vi "Measurement-IN.vi"(1 "Ctl Refnum 2":refnum<vi>, 2 "Ctl Refnum":refnum<vi>, 8 "error in (no error)":errorcluster, 9 "BSFR":refnum<file>, 10 "Cluster 2":T3, 11 "测试时间":dbl) -> (7 "Cluster":T1)   [LabVIEW 2017]
uses:
  <vilib>/Instr/_visa.llb/VISA Configure Serial Port (Instr).vi
panel:
  out "电抗":dbl
  out "电阻":dbl
  in  "Cluster 3":T2
  in  "高温&低温":u16(ring) items=["低温", "高温"]
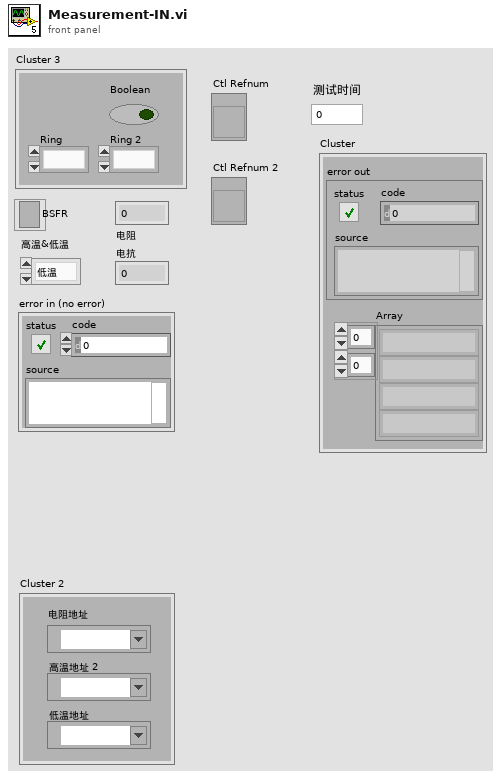
[diagram p1: front panel]
types:
  T1 = cluster{"Array":string[][], "error out":errorcluster}
  T2 = cluster{"Boolean":bool, "Ring":u16, "Ring 2":u16}
  T3 = cluster{"电阻地址":refnum<visa-resource-name>, "低温地址":refnum<visa-resource-name>, "高温地址 2":refnum<visa-resource-name>}
  T4 = cluster{"Array 2":string[][], "error out":errorcluster}
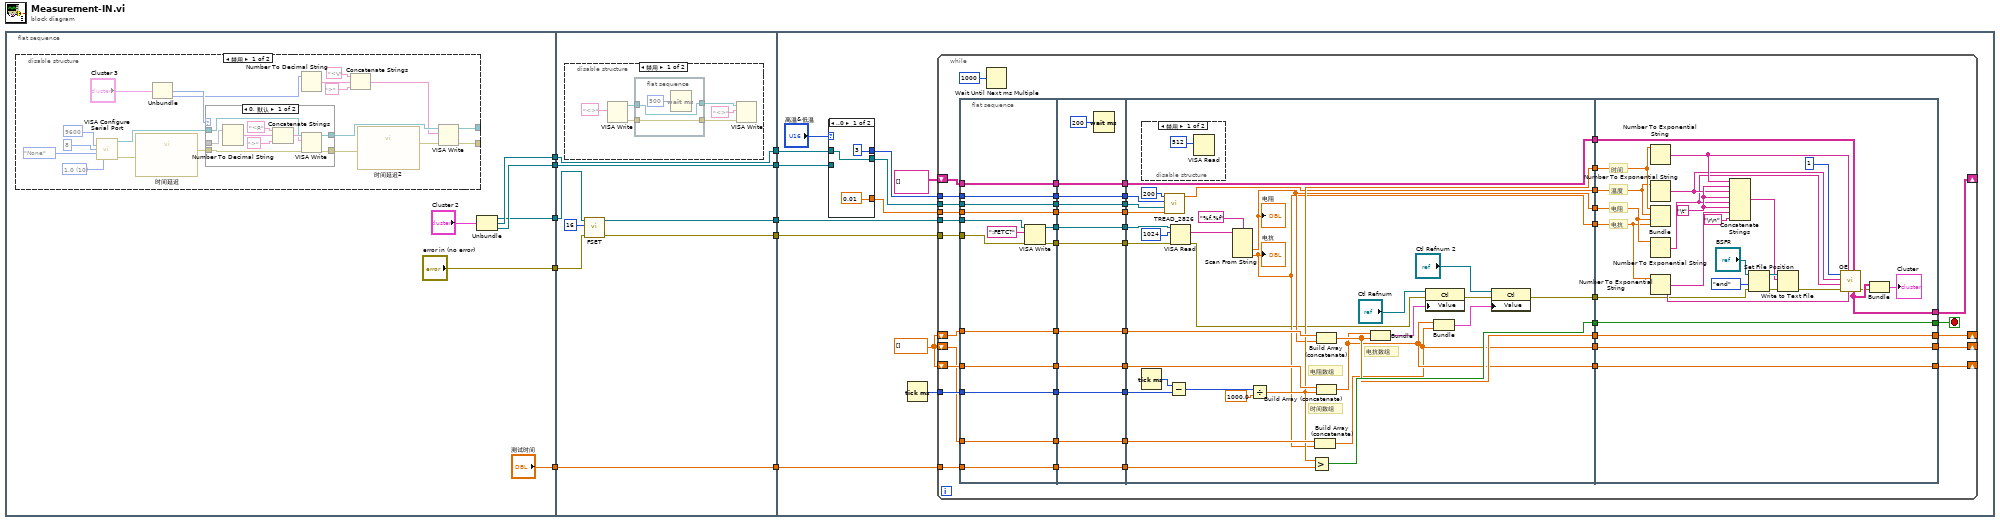
[diagram p0: block diagram]
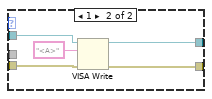
[diagram p2: hidden frame]
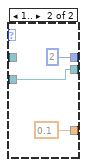
[diagram p5: hidden frame]
diagram:
  n1 = flat-sequence {
    tunnel: ["测试时间"] -> w9
    tunnel: [w15] -> w5
    tunnel: [w14] -> w4
    tunnel: [w11] -> w2
    tunnel: ["error in (no error)"] -> w1
    tunnel: [w57] -> w10
    tunnel: w9 -> [w57]
    tunnel: [w52] -> w8
    tunnel: [w56] -> w7
    tunnel: [w55] -> w6
    tunnel: w5 -> [w56]
    tunnel: w4 -> [w55]
    tunnel: [w50] -> w3
    tunnel: w2 -> [w53]
    tunnel: w1 -> [w51]
    tunnel: w10 -> [w72]
    tunnel: w8 -> [w71]
    tunnel: w7 -> [w70]
    tunnel: w6 -> [w69]
    tunnel: w3 -> [w68]
    frame #0 {
      n2 = disable-structure shown="禁用" {
        disable-tunnel: [w20 _] -> _
        disable-tunnel: [w19 _] -> _
        frame Disabled {
          w32 = u16 10 items=["1.0"=10, "1.5"=15, "2.0"=20] ("stop bits (10: 1 bit)")
          n3 = call-poly "VISA Configure Serial Port"("baud rate (9600)"=u32 9600, "data bits (8)"=u16 8, "parity (0:none)"=enum16{"None", "Odd", "Even", "Mark", "Space"}."None", "stop bits (10: 1 bit)"=w32) -> ("VISA resource name out"=w30:refnum<visa-resource-name>, "error out"=w24:errorcluster)  [unwired: 10 in]
          n4 = call "时间延迟"("error in (no error)"=w24) -> ("error out"=w23:errorcluster)  [unwired: 10 in]
          n5 = Unbundle("Cluster 3") -> ("Ring"=w18:u16, "Ring 2"=w17:u16)  [unwired: 1 out]
          n6 = case shown="0, 默认" w18 {
            tunnel: w30 -> [w44 w49]
            tunnel: _ -> [w41 _]
            tunnel: w23 -> [w38 w47]
            tunnel: [w37 w46] -> w29
            tunnel: [w36 w45] -> w21
            frame 0, Default {
              n7 = Number To Decimal String(number=w41) -> (decimal integer string=w40:string)  [unwired: 1 in]
              n8 = Concatenate Strings("<R" ("字符串"), w40, ">" ("字符串")) -> (w39:string)
              n9 = VISA Write(VISA resource name=w44, write buffer=w39, error in (no error)=w38) -> (VISA resource name out=w37:refnum<visa-resource-name>, error out=w36:errorcluster)  [unwired: 1 out]
            }
            frame 1 {
              n10 = VISA Write(VISA resource name=w49, write buffer="<A>" ("写入缓冲区"), error in (no error)=w47) -> (VISA resource name out=w46:refnum<visa-resource-name>, error out=w45:errorcluster)  [unwired: 1 out]
            }
          }
          n11 = Number To Decimal String(number=w17) -> (decimal integer string=w26:string)  [unwired: 1 in]
          n12 = Concatenate Strings("<V" ("字符串"), w26, ">" ("字符串")) -> (w25:string)
          n13 = call "时间延迟2"("error in (no error)"=w21) -> ("error out"=w22:errorcluster)  [unwired: 10 in]
          n14 = VISA Write(VISA resource name=w29, write buffer=w25, error in (no error)=w22) -> (VISA resource name out=w20:refnum<visa-resource-name>, error out=w19:errorcluster)  [unwired: 1 out]
        }
        frame Enabled {
        }
      }
      n15 = Unbundle("Cluster 2") -> ("电阻地址"=w11:refnum<visa-resource-name>, "低温地址"=w15:refnum<visa-resource-name>, "高温地址 2"=w14:refnum<visa-resource-name>)
    }
    frame #1 {
      n16 = disable-structure shown="禁用" {
        frame Disabled {
          n17 = VISA Write(write buffer="<>" ("写入缓冲区")) -> (VISA resource name out=w62:refnum<visa-resource-name>, error out=w60:errorcluster)  [unwired: 2 in, 1 out]
          n18 = flat-sequence {
            tunnel: w62 -> [w65]
            tunnel: [w65] -> w61
            tunnel: w60 -> [w64]
            tunnel: [w64] -> w59
            frame #0 {
              n19 = Wait (ms)(milliseconds to wait=u32 500 ("等待时间（毫秒）")) -> ()  [unwired: 1 out]
            }
          }
          n20 = VISA Write(VISA resource name=w61, write buffer="<>" ("写入缓冲区"), error in (no error)=w59) -> ()  [unwired: 3 out]
        }
        frame Enabled {
        }
      }
      n21 = call "FSET.vi"("error in (no error)"=w51, "Function (0: Cp-D)"=16, "VISA resource name"=w53) -> ("error out"=w50:errorcluster, "VISA resource name out"=w52:refnum<visa-resource-name>)  [unwired: 7 in]
    }
    frame #2 {
      w77 = dbl[] []
      n22 = case shown="..0" "高温&低温" {
        tunnel: [w79 w82] -> w75
        tunnel: [3 2] -> w74
        tunnel: [0.01 0.1] -> w73
        tunnel: w70 -> [w79 _]
        tunnel: w69 -> [_ w82]
        frame ..0 {
        }
        frame 1.. {
        }
      }
      n23 = Tick Count (ms)() -> (millisecond timer value=w78:u32)
      n24 = while {
        tunnel: w78 -> [w133]
        shift-right: [w126] -> _
        shift-left: w77 -> [w131]
        shift-right: [w127] -> _
        shift-left: w77 -> [w130]
        shift-right: [w128] -> _
        shift-left: w77 -> [w129]
        tunnel: w75 -> [w117]
        tunnel: w74 -> [w116]
        tunnel: w73 -> [w115]
        tunnel: w72 -> [w113]
        tunnel: w71 -> [w112]
        tunnel: w68 -> [w111]
        shift-right: [w89] -> _
        shift-left: string[][] [] -> [w85]
        stop <- w132 stop-if-true
        n25 = flat-sequence {
          tunnel: w111 -> [w135]
          tunnel: w113 -> [w140]
          tunnel: w112 -> [w138]
          tunnel: w115 -> [w141]
          tunnel: w116 -> [w142]
          tunnel: w117 -> [w143]
          tunnel: w129 -> [w144]
          tunnel: w130 -> [w145]
          tunnel: w131 -> [w146]
          tunnel: w133 -> [w147]
          tunnel: [w147] -> w110
          tunnel: [w146] -> w108
          tunnel: [w145] -> w106
          tunnel: [w144] -> w104
          tunnel: [w143] -> w102
          tunnel: [w142] -> w100
          tunnel: [w141] -> w98
          tunnel: [w137] -> w96
          tunnel: [w140] -> w94
          tunnel: [w136] -> w92
          tunnel: [w134] -> w86
          tunnel: w85 -> [w134]
          tunnel: w110 -> [w159]
          tunnel: [w159] -> w109
          tunnel: w108 -> [w158]
          tunnel: [w158] -> w107
          tunnel: w106 -> [w157]
          tunnel: [w157] -> w105
          tunnel: w104 -> [w156]
          tunnel: [w156] -> w103
          tunnel: w102 -> [w155]
          tunnel: [w155] -> w101
          tunnel: w100 -> [w154]
          tunnel: [w154] -> w99
          tunnel: w98 -> [w153]
          tunnel: [w153] -> w97
          tunnel: w96 -> [w152]
          tunnel: [w152] -> w95
          tunnel: w94 -> [w151]
          tunnel: [w151] -> w93
          tunnel: w92 -> [w150]
          tunnel: [w150] -> w91
          tunnel: [w148] -> w87
          tunnel: w86 -> [w148]
          tunnel: [w188] -> w125
          tunnel: [w163] -> w124
          tunnel: [w160] -> w123
          tunnel: [w162] -> w122
          tunnel: [w176] -> w121
          tunnel: [w175] -> w120
          tunnel: [w184] -> w119
          tunnel: [w161] -> w118
          tunnel: [w179] -> w114
          tunnel: w109 -> [w191]
          tunnel: w107 -> [w187]
          tunnel: w105 -> [w186]
          tunnel: w103 -> [w185]
          tunnel: w101 -> [w183]
          tunnel: w99 -> [w181]
          tunnel: w97 -> [w180]
          tunnel: w95 -> [w166]
          tunnel: w93 -> [w178]
          tunnel: w91 -> [w165]
          tunnel: [w164] -> w88
          tunnel: w87 -> [w164]
          tunnel: [w215] -> w132
          tunnel: w125 -> [w215]
          tunnel: [w214] -> w128
          tunnel: w124 -> [w214]
          tunnel: [w213] -> w127
          tunnel: w123 -> [w213]
          tunnel: [w212] -> w126
          tunnel: w122 -> [w212]
          tunnel: w121 -> [w206]
          tunnel: w120 -> [w205]
          tunnel: w119 -> [w208]
          tunnel: w118 -> [w196]
          tunnel: w114 -> [w207]
          tunnel: [w197] -> w89
          tunnel: w88 -> [w199]
          frame #0 {
            n26 = VISA Write(VISA resource name=w138, write buffer=":FETC?", error in (no error)=w135) -> (VISA resource name out=w137:refnum<visa-resource-name>, error out=w136:errorcluster)  [unwired: 1 out]
          }
          frame #1 {
            n27 = Wait (ms)(milliseconds to wait=u32 200 ("等待时间（毫秒）")) -> ()  [unwired: 1 out]
          }
          frame #2 {
            # "电抗数组"
            # "电阻数组"
            # "时间数组"
            n28 = disable-structure shown="禁用" {
              frame Disabled {
                n29 = VISA Read(byte count=u32 512 ("字节总数")) -> ()  [unwired: 2 in, 4 out]
              }
              frame Enabled {
              }
            }
            n30 = Tick Count (ms)() -> (millisecond timer value=w192:u32)
            n31 = call "TREAD_2826.vi"("Unknown Param 2"=w180, "VISA resource name"=w183, "Address No."=w181, "Unknown Param"=200) -> ("PV"=w179:dbl)  [unwired: 3 out]
            n32 = Subtract(x=w192, y=w191) -> (x-y=w190:u32)
            n33 = VISA Read(VISA resource name=w166, byte count=1024, error in (no error)=w165) -> (read buffer=w168:string, error out=w167:errorcluster)  [unwired: 2 out]
            n34 = Scan From String(format string="%f,%f" ("格式字符串"), input string=w168) -> (output 1=w176:dbl, output 2=w175:dbl)  [unwired: 4 in, 3 out]
            "电阻" <- w176
            "电抗" <- w175
            n35 = Divide(x=w190, y=1000.0) -> (x/y=w184:dbl)
            n36 = Greater?(x=w184, y=w178) -> (0:w188:bool)
            n37 = Build Array (concatenate)(w186, w175) -> (w160:dbl[])
            n38 = Build Array (concatenate)(w185, w176) -> (w163:dbl[])
            n39 = Build Array (concatenate)(w187, w184) -> (w162:dbl[])
            n40 = Bundle(w162, w163) -> (w171:cluster{dbl[], dbl[]})  [unwired: 1 in]
            n41 = property class="Ctl"(reference="Ctl Refnum", error in=w167, "Value"=w171) -> (error out=w172:errorcluster)  [unwired: 1 out]
            n42 = Bundle(w162, w160) -> (w170:cluster{dbl[], dbl[]})  [unwired: 1 in]
            n43 = property class="Ctl"(reference="Ctl Refnum 2", error in=w172, "Value"=w170) -> (error out=w161:errorcluster)  [unwired: 1 out]
          }
          frame #3 {
            w209 = "\t"
            # "温度"
            # "电抗"
            # "电阻"
            # "时间"
            n44 = Number To Exponential String(number=w208) -> (E-format string=w203:string)  [unwired: 3 out]
            n45 = Number To Exponential String(number=w207) -> (E-format string=w202:string)  [unwired: 3 out]
            n46 = Bundle(w208, "PV"=w207, "电阻"=w206, "电抗"=w205) -> ()  [unwired: 1 in, 1 out]
            n47 = Number To Exponential String(number=w206) -> (E-format string=w201:string)  [unwired: 3 out]
            n48 = Number To Exponential String(number=w205) -> (E-format string=w200:string)  [unwired: 1 in, 2 out]
            n49 = Concatenate Strings(w203, w209, w202, w209, w201, w209, w200, "\r\n") -> (w217:string)
            n50 = Set File Position(refnum="BSFR", from (0:start)=enum16{"start", "end", "current"}."end" ("自（0:起始）"), error in=w196) -> (refnum out=w219:refnum<file>, error out=w216:errorcluster)  [unwired: 1 out]
            n51 = Write to Text File(file (use dialog)=w219, text=w217, error in=w216) -> (error out=w194:errorcluster)  [unwired: 3 out]
            n52 = call "OE.vi"("Array"=w199, "String 4"=w200, "String"=w203, "error in (no error)"=w194, "String 3"=w201, "String 2"=w202, "Numeric"=1) -> ("error out"=w195:errorcluster, "Array 2"=w197:string[][])  [unwired: 2 in, 1 out]
            n53 = Bundle("Array 2"=w197, "error out"=w195) -> (→"Cluster":T4)  [unwired: 1 in]
          }
        }
        n54 = Wait Until Next ms Multiple(millisecond multiple=u32 1000 ("毫秒倍数")) -> ()  [unwired: 1 out]
      }
    }
  }
